vi "Set Clip Plane.vi"   [LabVIEW 2017, in "NI_3D Picture Control.lvlib"]
doc: "Defines the plane beyond which LabVIEW clips, or does not render, surfaces in a scene."
uses:
  <vilib>/picture/3D Picture Control/NI_3D Picture Control.lvlib
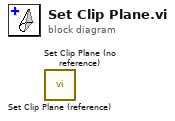
[diagram p0: block diagram]
diagram:
  n1 = call <vilib>:"Set Clip Plane (reference).vi"() -> ()  [unwired: 9 in, 3 out]
  n2 = call <vilib>:"Set Clip Plane (no reference).vi"() -> ()  [unwired: 10 in, 2 out]
